vi "Human.Execute.vi"(8 "error in (no error)":errorcluster) -> (0 "error out":errorcluster)   [LabVIEW 2020]
doc: "Execute for Human\n\ninput:\n error in (cluster)\n\noutput:\n error out (cluster)"
uses:
  <vilib>/Rock Robotics/WPI/Joystick/XBox Axes Indexer.ctl
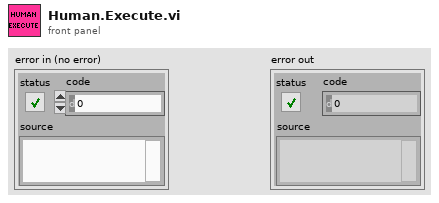
[diagram p1: front panel]
types:
  T1 = typedef "XBox Axes Indexer.ctl" = enum16{"Left X", "Left Y", "Left Trigger", "Right Trigger", "Right X", "Right Y"}
  T2 = typedef "WPI_JoystickDevRef.ctl" = cluster{"Device":T3}
  T3 = typedef "WPI_JoystickDeviceEnum.ctl" = enum16{"USB 0", "USB 1", "USB 2", "USB 3", "USB 4", "USB 5"}
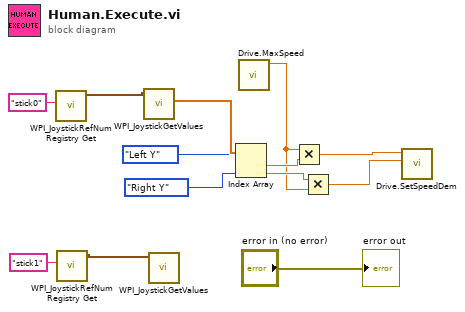
[diagram p0: block diagram]
diagram:
  n1 = call <vilib>:"WPI_JoystickRefNum Registry Get.vi"("refnum name"="stick0") -> ("JoystickDevRef"=w11:T2)  [unwired: 9 in, 1 out]
  n2 = call <vilib>:"WPI_JoystickRefNum Registry Get.vi"("refnum name"="stick1") -> ("JoystickDevRef"=w10:T2)  [unwired: 9 in, 1 out]
  n3 = call <vilib>:"WPI_JoystickGetValues.vi"("JoystickDevRef"=w11) -> ("Axes"=w9:dbl[])  [unwired: 6 in, 4 out]
  n4 = call <vilib>:"WPI_JoystickGetValues.vi"("JoystickDevRef"=w10) -> ()  [unwired: 6 in, 5 out]
  n5 = Index Array(array=w9, index #1=XBox_Axes_Indexer."Left Y" ("XBox Axes"), index #2=XBox_Axes_Indexer."Right Y" ("XBox Axes")) -> (element #1=w5:dbl, element #2=w6:dbl)
  n6 = call "Drive.MaxSpeed.vi"() -> ("Max Speed (ft/sec)"=w4:dbl)  [unwired: 11 in]
  n7 = Multiply(x=w4, y=w5) -> (x*y=w3:dbl)
  n8 = Multiply(x=w6, y=w4) -> (x*y=w2:dbl)
  n9 = call "Drive.SetSpeedDem.vi"("RSpeedDemand (ft/s)"=w2, "LSpeedDemand (ft/s)"=w3) -> ()  [unwired: 10 in]
  "error out" <- "error in (no error)"
